vi "HTS_WRITE_COMMAND.vi"(8 "Error IN":errorcluster, 10 "Command":string, 11 "HTS PORT IN":refnum<visa-resource-name>="HTS") -> (0 "Error OUT":errorcluster, 2 "RESPONSE":string[](array[string]), 3 "HTS PORT OUT":refnum<visa-resource-name>)   [LabVIEW 2013]
uses:
  <vilib>/Instr/_visa.llb/VISA Configure Serial Port (Instr).vi
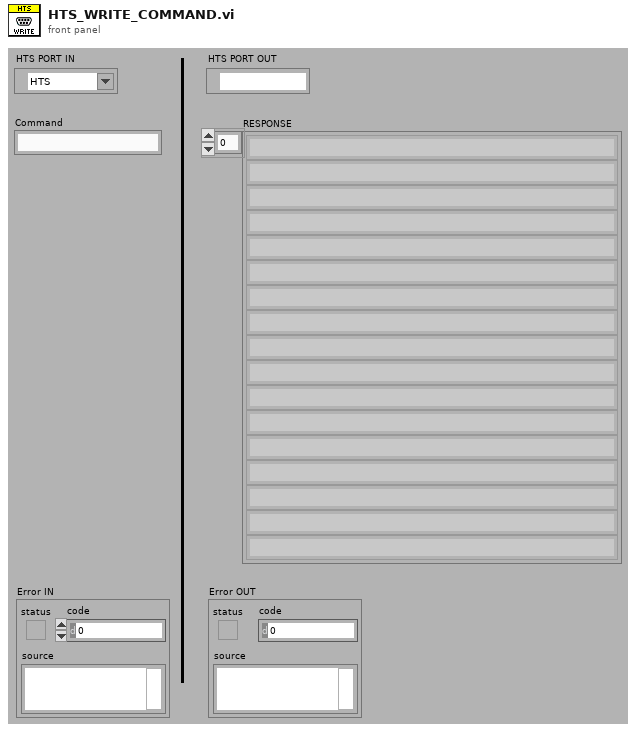
[diagram p1: front panel]
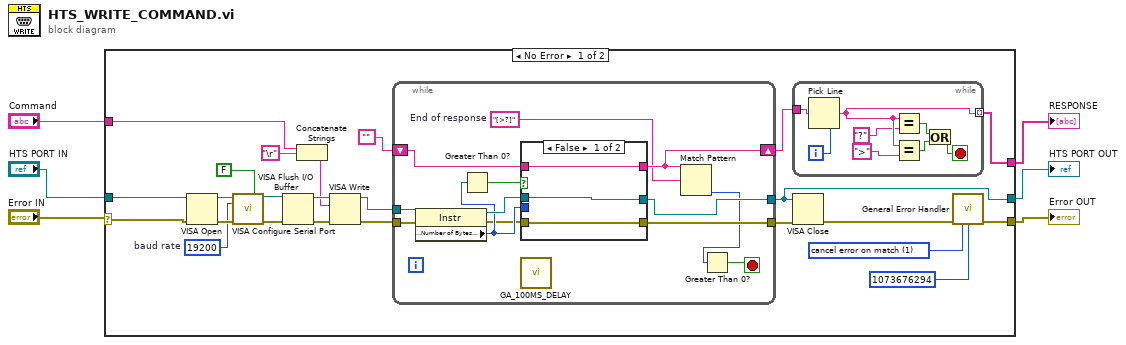
[diagram p0: block diagram]
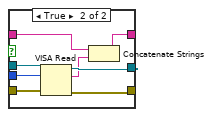
[diagram p2: hidden frame]
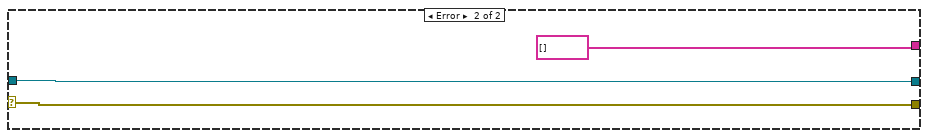
[diagram p3: hidden frame]
diagram:
  n1 = case shown="No Error" "Error IN" {
    selector: "Error IN" -> [w7 w63]
    tunnel: "HTS PORT IN" -> [w24 w64]
    tunnel: [w19 w64] -> w5
    tunnel: "Command" -> [w8 _]
    tunnel: [w14 string[] []] -> w3
    tunnel: [w10 w63] -> w2
    frame No Error {
      w13 = 1 items=["no exception", "cancel error on match", "set error on match"] ("[exception action] (none:0)")
      w18 = u32 19200  # baud rate
      n2 = VISA Open(error in (no error)=w7, VISA resource name=w24) -> (VISA resource name=w28:refnum<visa-resource-name>, error out=w27:errorcluster)  [unwired: 3 out]
      n3 = call-poly "VISA Configure Serial Port"("VISA resource name"=w28, "Enable Termination\nChar (T)"=FALSE ("Enable Termination\nChar (T)"), "baud rate (9600)"=w18, "error in (no error)"=w27) -> ("VISA resource name out"=w29:refnum<visa-resource-name>, "error out"=w30:errorcluster)  [unwired: 3 in, 7 out]
      n4 = VISA Flush I/O Buffer(VISA resource name=w29, error in (no error)=w30) -> (VISA resource name out=w26:refnum<visa-resource-name>, error out=w25:errorcluster)  [unwired: 1 out]
      n5 = Concatenate Strings(w8, "\r") -> (w16:string)
      n6 = VISA Write(VISA resource name=w26, write buffer=w16, error in (no error)=w25) -> (VISA resource name out=w20:refnum<visa-resource-name>, error out=w22:errorcluster)  [unwired: 1 out]
      n7 = while {
        tunnel: w20 -> [w51]
        tunnel: [w49] -> w19
        tunnel: [w45] -> w21
        shift-right: [w43] -> w15
        shift-left: "" -> [w44]
        tunnel: w22 -> [w39]
        stop <- w42 stop-if-true
        w40 = "[>?]"  # End of response
        n8 = property class="Instr"(reference=w51, error in=w39) -> (reference out=w50:refnum<visa-resource-name>, error out=w46:errorcluster, "Serial Settings:Number of Bytes at Serial Port"=w47:u32)
        n9 = Greater Than 0?(x=w47) -> (x > 0?=w48:bool)
        n10 = case shown="False" w48 {
          tunnel: w50 -> [w54 w62]
          tunnel: [w54 w61] -> w49
          tunnel: w47 -> [_ w60]
          tunnel: w46 -> [w53 w59]
          tunnel: [w53 w58] -> w45
          tunnel: w44 -> [w52 w57]
          tunnel: [w52 w55] -> w43
          frame False {
          }
          frame True {
            n11 = VISA Read(VISA resource name=w62, byte count=w60, error in (no error)=w59) -> (VISA resource name out=w61:refnum<visa-resource-name>, read buffer=w56:string, error out=w58:errorcluster)  [unwired: 1 out]
            n12 = Concatenate Strings(w57, w56) -> (w55:string)
          }
        }
        n13 = call "GA_100MS_DELAY.vi"() -> ()  [unwired: 1 in, 11 out]
        n14 = Match Pattern(string=w43, regular expression=w40) -> (offset past match=w41:i32)  [unwired: 4 out]
        n15 = Greater Than 0?(x=w41) -> (x > 0?=w42:bool)
      }
      n16 = while {
        tunnel: w15 -> [w37]
        tunnel: [w32] -> w14 mode=indexing
        i -> [w38]
        stop <- w35 stop-if-true
        n17 = Pick Line(multi-line string=w37, line index=w38) -> (output string=w32:string)  [unwired: 1 out]
        n18 = Equal?(x=w32, y="?" ("regular expression")) -> (x = y?=w34:bool)
        n19 = Equal?(x=w32, y=">" ("regular expression")) -> (x = y?=w33:bool)
        n20 = Or(x=w34, y=w33) -> (x .or. y?=w35:bool)
      }
      n21 = VISA Close(VISA resource name=w19, error in (no error)=w21) -> (error out=w11:errorcluster)
      n22 = call <vilib>:"General Error Handler.vi"("error in (no error)"=w11, "[exception action] (none:0)"=w13, "[exception code]"=1073676294) -> ("error out"=w10:errorcluster)  [unwired: 1 in, 11 out]
    }
    frame Error {
    }
  }
  "Error OUT" <- w2
  "RESPONSE" <- w3
  "HTS PORT OUT" <- w5
